vi "交通灯控制系统.vi"() -> ()   [LabVIEW 2024]
panel:
  in  "白天\n\n黑夜":bool caption="布尔 7"
  in  "停止":bool
  out "Cluster 4":T1 caption="簇"
  out "Cluster 3":T1 caption="簇"
  out "Cluster 2":T1 caption="簇"
  out "Cluster":T1 caption="簇"
  out "布尔 6":bool
  out "布尔 5":bool
  out "布尔 4":bool
  out "布尔 3":bool
  out "布尔 2":bool
  out "布尔":bool
  # "北"
  # "西"
  # "东"
  # "南"
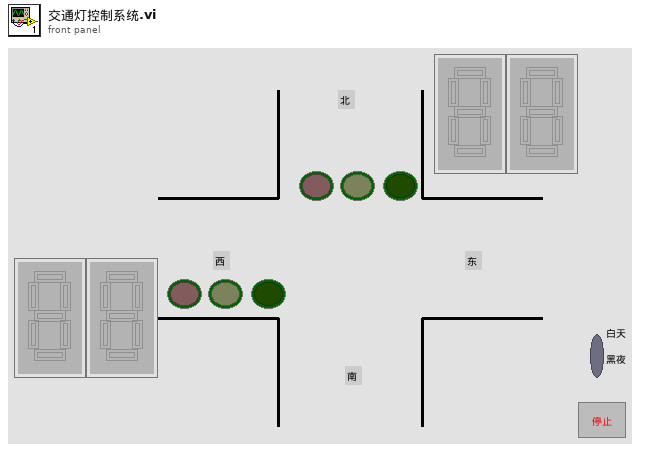
[diagram p1: front panel]
types:
  T1 = cluster{"布尔":bool, "布尔 5":bool, "布尔 4":bool, "布尔 2":bool, "布尔 6":bool, "布尔 7":bool, "布尔 3":bool}
  T2 = cluster{"[0]":bool, "[1]":bool, "[2]":bool, "[3]":bool, "[4]":bool, "[5]":bool}
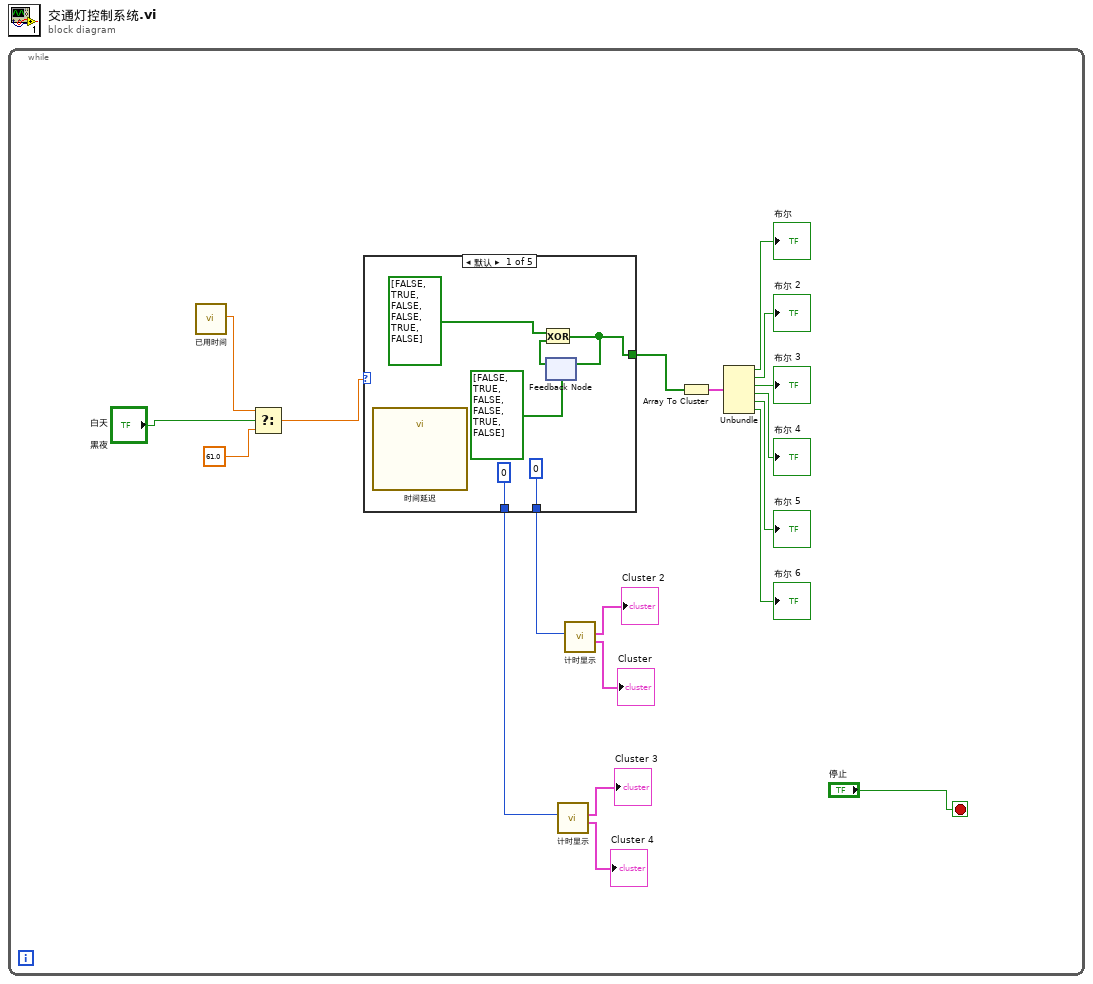
[diagram p0: block diagram]
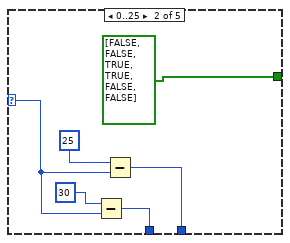
[diagram p2: hidden frame]
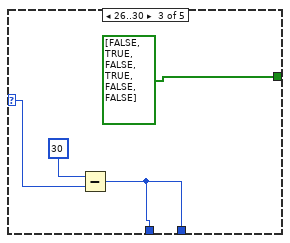
[diagram p3: hidden frame]
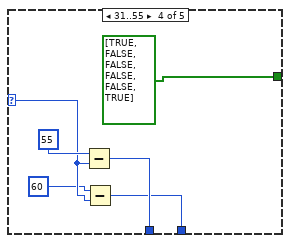
[diagram p4: hidden frame]
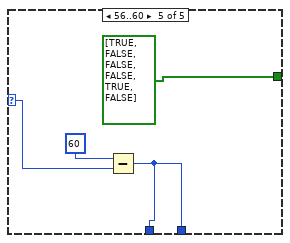
[diagram p5: hidden frame]
diagram:
  n1 = while {
    stop <- "停止" stop-if-true
    n2 = call "已用时间"() -> ("Elapsed Time (s)"=w3:dbl)  [unwired: 12 in, 7 out]
    n3 = Select(t=w3, s="白天\n\n黑夜", f=61.0) -> (s? t:f=w2:dbl)
    n4 = case shown="默认" w2 {
      selector: w2 -> [_ w27 w33 w37 w44]
      tunnel: [w21 bool[] [FALSE, FALSE, TRUE, TRUE, FALSE, FALSE] bool[] [FALSE, TRUE, FALSE, TRUE, FALSE, FALSE] bool[] [TRUE, FALSE, FALSE, FALSE, FALSE, TRUE] bool[] [TRUE, FALSE, FALSE, FALSE, TRUE, FALSE]] -> w14
      tunnel: [0 w29 w32 w38 w42] -> w6
      tunnel: [0 ("数值") w28 w32 w39 w42] -> w5
      frame Default {
        n5 = call "时间延迟"() -> ()  [unwired: 11 in, 1 out]
        n6 = feedback #1(bool[] [FALSE, TRUE, FALSE, FALSE, TRUE, FALSE]) -> (w20:bool[])
        n7 = Exclusive Or(1:w20, 2:bool[] [FALSE, TRUE, FALSE, FALSE, TRUE, FALSE]) -> (0:w21:bool[])
        n8 = feedback-in #1(w21) -> ()
      }
      frame 0..25 {
        n9 = Subtract(x=30, y=w27) -> (x-y=w28:i32)
        n10 = Subtract(x=25, y=w27) -> (x-y=w29:i32)
      }
      frame 26..30 {
        n11 = Subtract(x=30, y=w33) -> (x-y=w32:i32)
      }
      frame 31..55 {
        n12 = Subtract(x=55, y=w37) -> (x-y=w39:i32)
        n13 = Subtract(x=60, y=w37) -> (x-y=w38:i32)
      }
      frame 56..60 {
        n14 = Subtract(x=60, y=w44) -> (x-y=w42:i32)
      }
    }
    n15 = call "计时显示.vi"("数值"=w5) -> ("Cluster"=→"Cluster 4":T1, "Cluster 2"=→"Cluster 3":T1)  [unwired: 9 in]
    n16 = call "计时显示.vi"("数值"=w6) -> ("Cluster"=→"Cluster":T1, "Cluster 2"=→"Cluster 2":T1)  [unwired: 9 in]
    n17 = Array To Cluster(array=w14) -> (cluster=w13:T2)
    n18 = Unbundle(w13) -> ("[0]"=→"布尔":bool, "[1]"=→"布尔 2":bool, "[2]"=→"布尔 3":bool, "[3]"=→"布尔 4":bool, "[4]"=→"布尔 5":bool, "[5]"=→"布尔 6":bool)
  }
